vi "MS Write.vi"(0 "VISA Refnum in":refnum<visa-resource-name>, 1 "Up":dbl, 2 "Ie":dbl, 3 "delay":u32=500, 4 "error in (no error)":errorcluster) -> (5 "error out":errorcluster, 6 "VISA Refnum out":refnum<visa-resource-name>)   [LabVIEW 2012]
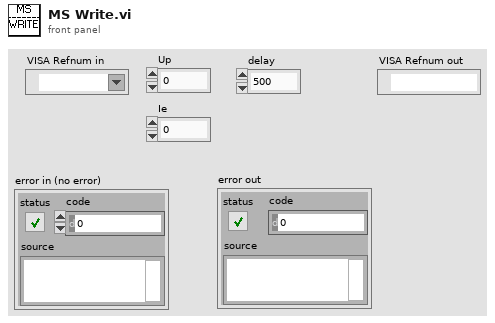
[diagram p1: front panel]
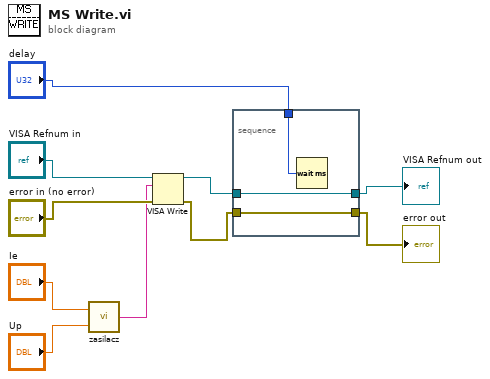
[diagram p0: block diagram]
diagram:
  n1 = call "zasilacz.vi"("Up"="Up", "Ie"="Ie") -> ("data string"=w6:string)
  n2 = VISA Write(VISA resource name="VISA Refnum in", write buffer=w6, error in (no error)="error in (no error)") -> (VISA resource name out=w5:refnum<visa-resource-name>, error out=w3:errorcluster)  [unwired: 1 out]
  n3 = stacked-sequence {
    tunnel: [w13] -> w4
    tunnel: w5 -> [w13]
    tunnel: w3 -> [w12]
    tunnel: [w12] -> w2
    tunnel: "delay" -> [w11]
    frame #0 {
      n4 = Wait (ms)(milliseconds to wait=w11) -> ()  [unwired: 1 out]
    }
  }
  "VISA Refnum out" <- w4
  "error out" <- w2
